vi "workspace.rid.vi"(8 "error in":errorcluster, 11 "Workspace in":refnum<class "Workspace.lvclass">) -> (0 "error out":errorcluster, 3 "Workspace out":refnum<class "Workspace.lvclass">)   [LabVIEW 2020, in "Workspace.lvclass"]
doc: "Returns the workspace's unique identifier (RID)."
uses:
  Workspace.lvclass
  Workspace.lvclass/Workspace.ctl
  client.lvlib
panel:
  out "out_needed out":u32
  out "rid":string
  in  "buf":string
  in  "cap":u32
  in  "out_needed":u32
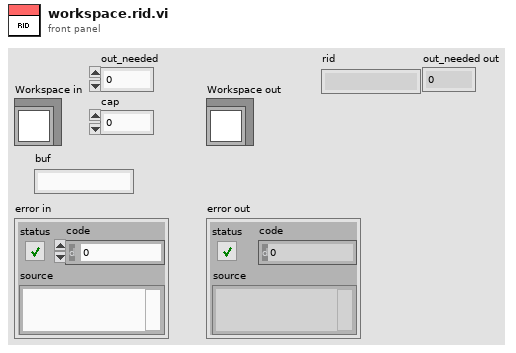
[diagram p1: front panel]
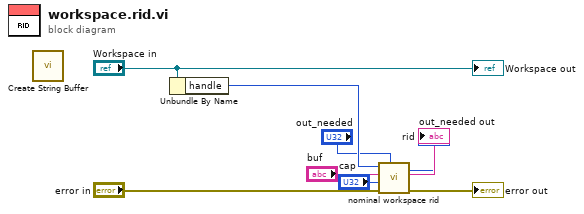
[diagram p0: block diagram]
diagram:
  n1 = call "Create String Buffer.vi"() -> ()  [unwired: 9 in, 3 out]
  n2 = Unbundle By Name("Workspace in") -> ("handle"=w7:i32)
  n3 = call "nominal workspace rid.vi"("out_needed"="out_needed", "error in (no error)"="error in", "cap"="cap", "buf"="buf", "workspace"=w7) -> ("error out"=→"error out":errorcluster, "buf out"=→"rid":string, "out_needed out"=→"out_needed out":u32)  [unwired: 3 in, 1 out]
  "Workspace out" <- "Workspace in"
